vi "MT Align To Ideal Symbols.vi"   [LabVIEW 2020, in "niDMT.lvlib"]
doc: "Locates the first occurrence of the ideal symbol timing instant in the matched filtered <B>input complex waveform</B>. It then applies phase-continuous resampling to align the first sample of the <B>input complex waveform</B> to the ideal symbol timing instant. The returned waveform is symbol-time aligned such that its first sample corresponds to the optimal (ideal) symbol instant."
uses:
  <vilib>/addons/Modulation/niDMT.lvlib
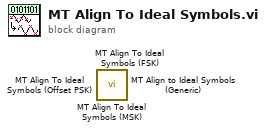
[diagram p0: block diagram]
diagram:
  n1 = call <vilib>:"MT Align To Ideal Symbols (MSK).vi"() -> ()  [unwired: 13 in, 3 out]
  n2 = call <vilib>:"MT Align To Ideal Symbols (FSK).vi"() -> ()  [unwired: 13 in, 3 out]
  n3 = call <vilib>:"MT Align To Ideal Symbols (Offset PSK).vi"() -> ()  [unwired: 12 in, 4 out]
  n4 = call <vilib>:"MT Align to Ideal Symbols (Generic).vi"() -> ()  [unwired: 13 in, 3 out]
